vi "Get Channels by Name.vi"(8 "error in (no error)":errorcluster, 11 "Sift Stream in":refnum<class "Sift Stream.lvclass">) -> (0 "error out":errorcluster, 1 "Channels":refnum<class "Channel.lvclass">[](array[class]), 3 "Sift Stream out":refnum<class "Sift Stream.lvclass">)   [LabVIEW 2024, in "Sift Stream.lvlib" / "Sift Stream.lvclass"]
uses:
  Sift Stream.lvclass
  Sift Stream.lvclass/Sift Stream.ctl
  <vilib>/FlexLogger/SDK/PluginSDK.lvlibp/PEFClasses/SDK/Consumer Channel/Consumer Channel.lvclass
  C:/Program Files/National Instruments/LabVIEW 2024/vi.lib/FlexLogger/SDK/PluginSDK.lvlibp/PEFClasses/SDK/Channel/Channel.lvclass
  C:/Program Files/National Instruments/LabVIEW 2024/vi.lib/FlexLogger/SDK/PluginSDK.lvlibp/PEFClasses/SDK/Consumer Channel/Consumer Channel.lvclass
  <vilib>/FlexLogger/SDK/PluginSDK.lvlibp/PEFClasses/SDK/Channel/Channel.lvclass
panel:
  in  "Stream Names":string[](array[string])
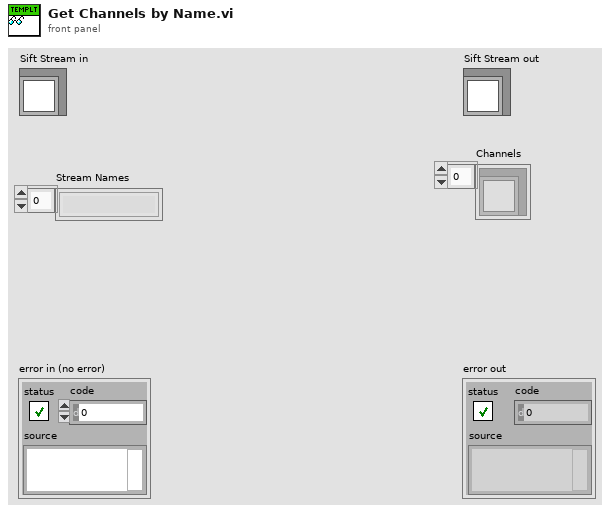
[diagram p1: front panel]
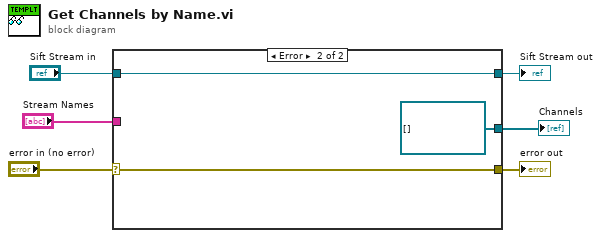
[diagram p0: block diagram]
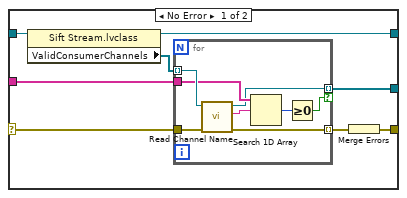
[diagram p2: hidden frame]
diagram:
  n1 = case shown="Error" "error in (no error)" {
    selector: "error in (no error)" -> [w10 w24]
    tunnel: [w7 w24] -> w2
    tunnel: [w13 w25] -> w4
    tunnel: "Sift Stream in" -> [w14 w25]
    tunnel: "Stream Names" -> [w11 _]
    tunnel: [w9 refnum<class "Consumer Channel.lvclass">[] []] -> w1
    frame No Error {
      n2 = property class="Sift Stream.lvclass"(reference=w14) -> (reference out=w13:refnum<class "Sift Stream.lvclass">, "ValidConsumerChannels"=w12:refnum<class "Consumer Channel.lvclass">[])  [unwired: 1 in, 1 out]
      n3 = for {
        tunnel: w12 -> [w22] mode=indexing
        tunnel: w11 -> [w19]
        tunnel: w10 -> [w21]
        tunnel: [w20] -> w8 mode=indexing
        tunnel: [w16] -> w9 mode=indexing if=w15
        n4 = call-dynamic "Read Channel Name.vi"("error in (no error)"=w21, "Channel in"=w22) -> ("error out"=w20:errorcluster, "Channel Name"=w18:string, "Channel out"=w16:refnum<class "Consumer Channel.lvclass">)  [unwired: 7 in]
        n5 = Search 1D Array(1D array=w19, element=w18) -> (index of element=w17:i32)  [unwired: 1 in]
        n6 = Greater Or Equal To 0?(x=w17) -> (x >= 0?=w15:bool)
      }
      n7 = Merge Errors(w8) -> (w7:errorcluster)
    }
    frame Error {
    }
  }
  "error out" <- w2
  "Sift Stream out" <- w4
  "Channels" <- w1
